vi "Run Solver.vi"(8 "error in (no error)":errorcluster, 11 "Solver VI":refnum<vi>) -> (0 "error out":errorcluster, 2 "Completed":bool, 3 "Run Time":dbl)   [LabVIEW 2024, in "Word Search Scorer.lvlib"]
uses:
  Word Search Scorer.lvlib
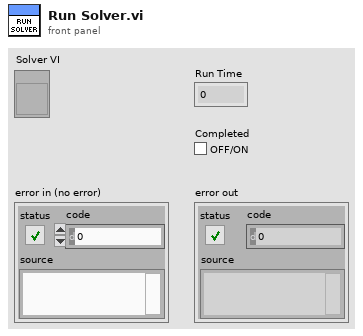
[diagram p1: front panel]
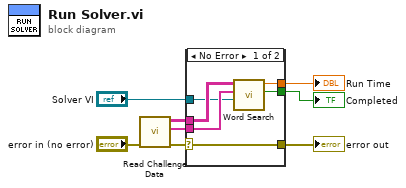
[diagram p0: block diagram]
diagram:
  n1 = call "Read Challenge Data.vi"("error in (no error)"="error in (no error)") -> ("error out"=w4:errorcluster, "Word List"=w6:string[], "Grid"=w7:string[][])  [unwired: 8 in]
  n2 = case shown="No Error" w4 {
    selector: w4 -> [w11 w15]
    tunnel: w7 -> [w14 _]
    tunnel: w6 -> [w13 _]
    tunnel: "Solver VI" -> [w12 _]
    tunnel: [w11 w15] -> w3
    tunnel: [w10 _] -> w2
    tunnel: [w9 _] -> w1
    frame No Error {
      n3 = call "Word Search.vi"("Solver VI"=w12, "Word List"=w13, "Word Search Grid"=w14) -> ("All Words Found"=w9:bool, "Execution Time"=w10:dbl)  [unwired: 7 in]
    }
    frame Error {
    }
  }
  "error out" <- w3
  "Run Time" <- w2
  "Completed" <- w1
